vi "ttm_stop_poller.vi"() -> ()   [LabVIEW 2011]
panel:
  out "error out":errorcluster
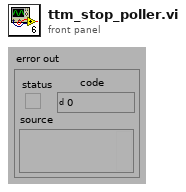
[diagram p1: front panel]
types:
  T1 = cluster{"Device ID":i32, "Device Name":string, "Device Type":i32}[]
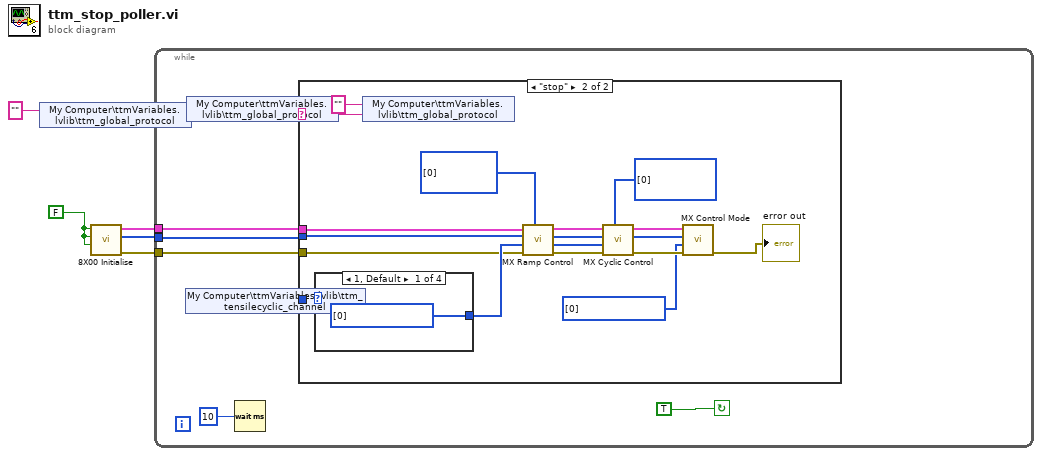
[diagram p0: block diagram]
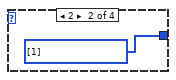
[diagram p3: hidden frame]
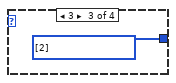
[diagram p4: hidden frame]
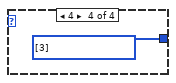
[diagram p5: hidden frame]
diagram:
  w5 = FALSE ("Create Console? (T)")
  n1 = shared-variable "My Computer\\ttmVariables.lvlib\\ttm_global_protocol"("" ("protocol")) -> ()  [unwired: 1 in, 1 out]
  n2 = call "8X00 Initialise.vi"("Reset?"=w5, "Create DVM? (T)"=w5, "Create Console? (T)"=w5) -> ("error out"=w2:errorcluster, "Axis Selector"=w3:i32[], "Axis Information"=w4:T1)  [unwired: 1 in, 1 out]
  n3 = while {
    tunnel: w4 -> [w11]
    tunnel: w3 -> [w12]
    tunnel: w2 -> [w10]
    stop <- TRUE continue-if-true
    n4 = shared-variable "My Computer\\ttmVariables.lvlib\\ttm_tensilecyclic_channel"() -> (w6:i32)  [unwired: 1 in, 1 out]
    n5 = shared-variable "My Computer\\ttmVariables.lvlib\\ttm_global_protocol"() -> (w8:string)  [unwired: 1 in, 1 out]
    n6 = Wait (ms)(milliseconds to wait=u32 10) -> ()  [unwired: 1 out]
    n7 = case shown="\"stop\"" w8 {
      tunnel: w12 -> [_ w26]
      tunnel: w11 -> [_ w25]
      tunnel: w10 -> [_ w27]
      tunnel: w6 -> [_ w29]
      frame "", Default {
      }
      frame "stop" {
        w13 = u16[] [0] items=["Channel 1", "Channel 2", "Channel 3", "Channel 4"] ("Control Modes")
        w19 = u16[] [0] items=["Stop", "Start or continue", "Hold", "Continue", "Finish current cycle & stop", "Smooth Stop", "Reserved", "Reserved", "Reserved", "Reserved", "Reserved", "Reserved", "Disable", "Enable", "Reserved", "Reserved", "Start/Continue swept waveform", "Dwell at swept frequency"] ("Cyclic Control")
        w20 = u16[] [0] items=["Stop", "Start or continue", "Hold", "Continue", "Return ramp to set level at fixed rate", "Reserved", "Reserved", "Start Random without demand hold", "Start Random with demand hold", "Prepare Random Start without demand hold", "Prepare Random Start with demand hold", "Unslave", "Reserved", "Reserved", "Start Sample Data Playback or Resume", "Prepare for Start of Sample Data", "Reserved", "Reserved", "Resume Playback", "Start an electromechanical frame return"] ("Ramp Control")
        n8 = case shown="1, Default" w29 {
          tunnel: [w30 w31 w32 w33] -> w28
          frame 1, Default {
            w30 = u16[] [0] items=["Channel 1", "Channel 2", "Channel 3", "Channel 4"] ("Choose channel to apply\nthe setpoint")
          }
          frame 2 {
            w31 = u16[] [1] items=["Channel 1", "Channel 2", "Channel 3", "Channel 4"] ("Choose channel to apply\nthe setpoint")
          }
          frame 3 {
            w32 = u16[] [2] items=["Channel 1", "Channel 2", "Channel 3", "Channel 4"] ("Choose channel to apply\nthe setpoint")
          }
          frame 4 {
            w33 = u16[] [3] items=["Channel 1", "Channel 2", "Channel 3", "Channel 4"] ("Choose channel to apply\nthe setpoint")
          }
        }
        n9 = shared-variable "My Computer\\ttmVariables.lvlib\\ttm_global_protocol"("" ("protocol")) -> ()  [unwired: 1 in, 1 out]
        n10 = call "MX Ramp Control.vi"("Ramp Control"=w20, "error in (no error)"=w27, "Channels In"=w28, "Axis Selector In"=w26, "Axis Information In"=w25) -> ("error out"=w21:errorcluster, "Channels Out"=w22:u16[], "Axis Selector Out"=w23:i32[], "Axis Information Out"=w24:T1)  [unwired: 2 in]
        n11 = call "MX Cyclic Control.vi"("Cyclic Control"=w19, "error in (no error)"=w21, "Channels"=w22, "Axis Selector"=w23, "Axis Information"=w24) -> ("error out"=w17:errorcluster, "Axis Selector out"=w14:i32[], "Axis Information out"=w16:T1)  [unwired: 2 in, 1 out]
        n12 = call "MX Control Mode.vi"("error in (no error)"=w17, "Control Modes"=w13, "Axis Selector"=w14, "Axis Information"=w16) -> ("error out"=→"error out":errorcluster)  [unwired: 2 in, 3 out]
      }
    }
  }
